vi "Query Cycle Progress.vi"(8 "error in (no error)":errorcluster, 10 "Cycle (0: Average Flow)":u16(ring) items=["Leak Check", "Purge", "Total"], 11 "VISA resource name":refnum<visa-resource-name>) -> (0 "error out":errorcluster, 2 "Seconds":dbl, 3 "VISA resource name out":refnum<visa-resource-name>)   [LabVIEW 2023, in "Fluke Molbox 1 Plus.lvlib"]
doc: "Queries the instrument on the progress of a specific cycle. This value is the amount of seconds remaining in the cycle."
uses:
  Fluke Molbox 1 Plus.lvlib
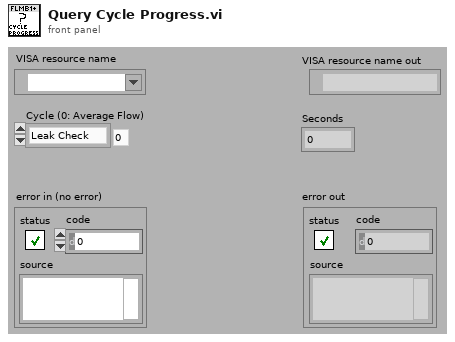
[diagram p1: front panel]
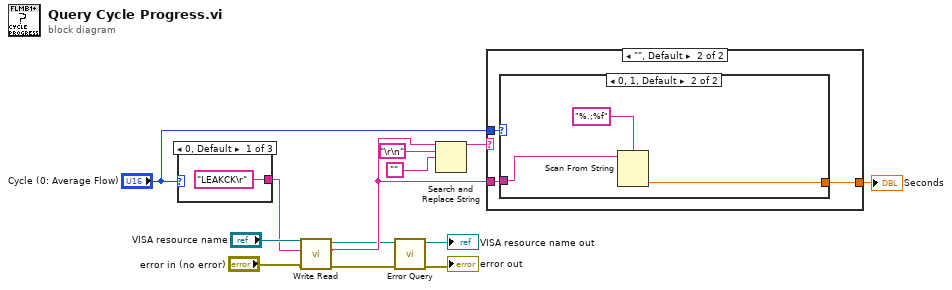
[diagram p0: block diagram]
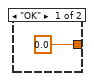
[diagram p2: hidden frame]
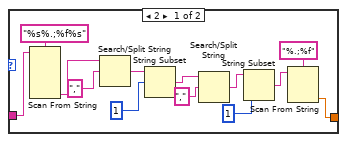
[diagram p3: hidden frame]
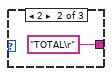
[diagram p4: hidden frame]
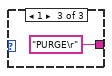
[diagram p5: hidden frame]
diagram:
  n1 = case shown="0, Default" "Cycle (0: Average Flow)" {
    tunnel: ["LEAKCK\r" "TOTAL\r" "PURGE\r"] -> w6
    frame 0, Default {
    }
    frame 2 {
    }
    frame 1 {
    }
  }
  n2 = call "Write Read.vi"("error in (no error)"="error in (no error)", "Write String"=w6, "VISA resource name"="VISA resource name") -> ("error out"=w3:errorcluster, "Read Response"=w5:string, "VISA resource name out"=w4:refnum<visa-resource-name>)  [unwired: 6 in]
  n3 = call "Error Query.vi"("error in (no error)"=w3, "VISA resource name"=w4) -> ("error out"=→"error out":errorcluster, "VISA resource name out"=→"VISA resource name out":refnum<visa-resource-name>)  [unwired: 6 in, 2 out]
  n4 = Search and Replace String(input string=w5, search string="\r\n" ("End of Line Constant"), replace string="" ("Empty String Constant")) -> (result string=w9:string)  [unwired: 5 in, 3 out]
  n5 = case shown="\"\", Default" w9 {
    tunnel: w5 -> [_ w20]
    tunnel: "Cycle (0: Average Flow)" -> [_ w19]
    tunnel: [0.0 w18] -> w12
    frame "OK" {
    }
    frame "", Default {
      n6 = case shown="0, 1, Default" w19 {
        tunnel: w20 -> [w33 w36]
        tunnel: [w22 w34] -> w18
        frame 2 {
          n7 = Scan From String(format string="%s%.;%f%s", input string=w33) -> (output 3=w28:string)  [unwired: 7 in, 3 out]
          n8 = Search/Split String(string=w28, search string/char (-)=",") -> (match + rest of string=w30:string)  [unwired: 1 in, 2 out]
          n9 = String Subset(string=w30, offset (0)=1) -> (substring=w24:string)  [unwired: 1 in]
          n10 = Search/Split String(string=w24, search string/char (-)=",") -> (match + rest of string=w26:string)  [unwired: 1 in, 2 out]
          n11 = String Subset(string=w26, offset (0)=1) -> (substring=w23:string)  [unwired: 1 in]
          n12 = Scan From String(format string="%.;%f", input string=w23) -> (output 1=w22:dbl)  [unwired: 3 in, 3 out]
        }
        frame 0, 1, Default {
          n13 = Scan From String(format string="%.;%f", input string=w36) -> (output 1=w34:dbl)  [unwired: 3 in, 3 out]
        }
      }
    }
  }
  "Seconds" <- w12
